vi "Core-Timer.vi"(7 "Ticks Begin In [ms]":u64, 8 "error in (no error)":errorcluster, 11 "Engine in":refnum<class "Engine.lvclass">) -> (0 "error out":errorcluster, 3 "Engine out":refnum<class "Engine.lvclass">, 5 "Ticks Begin Out [ms]":u64)   [LabVIEW 2020, in "GLF.lvlib" / "Engine.lvclass"]
uses:
  Engine.lvclass
  Engine.lvclass/Engine.ctl
  <vilib>/Saukko/LV SDL3/Sources/SDL3/Timer/Timer.lvlib
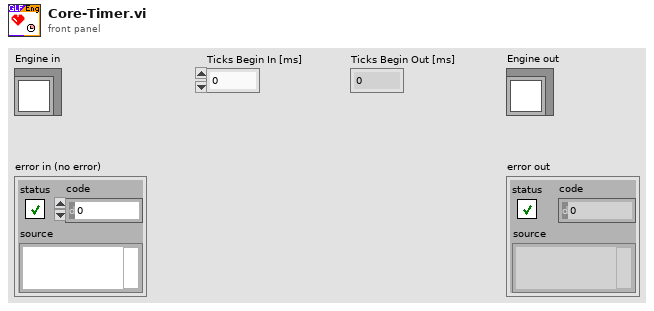
[diagram p1: front panel]
types:
  T1 = typedef "GLF.lvlib/Engine.lvclass/DVR--cluster.ctl" = cluster{"CMD Queue":T2, "Config":T3, "Ctxt":T5, "Metrics":T6, "Debug":T7, "ID To Window":map{T9, refnum<class "Window.lvclass">}, "Window To Handle":map{refnum<class "Window.lvclass">, i64}, "Event Interface":refnum<class "EngineEventInterface.lvclass">}
  T2 = typedef "GLF.lvlib/Engine.lvclass/Command--queue.ctl" = refnum<queue>
  T3 = typedef "GLF.lvlib/Engine.lvclass/Config--cluster.ctl" = cluster{"Quit On Last Window Closed":bool, "VSync":T4, "FPS Target":dbl}
  T4 = typedef "GLF.lvlib/Engine.lvclass/VSync--enum.ctl" = enum16{"Disabled", "Enabled", "Adaptative"}
  T5 = typedef "GLF.lvlib/Engine.lvclass/Context--cluster.ctl" = cluster{"VSync Enabled":bool}
  T6 = typedef "GLF.lvlib/Engine.lvclass/Metrics--cluster.ctl" = cluster{"Uptime [ms]":u64, "Loop Time [ms]":u64, "Timer [ns]":u64, "Poll Events [ns]":u64, "Dequeue CMD [ns]":u64, "Update Layout [ns]":u64, "Render [ns]":u64}
  T7 = typedef "GLF.lvlib/Engine.lvclass/Debug--cluster.ctl" = cluster{"Unhandled Events":map{T8, u64}}
  T8 = typedef "SDL3.lvlib/Events.lvlib/EventType--enum.ctl" = enum16{"LV_NONE", "LV_UNSUPPORTED", "SDL_EVENT_QUIT", "SDL_EVENT_LOCALE_CHANGED", "SDL_EVENT_SYSTEM_THEME_CHANGED", "SDL_EVENT_DISPLAY_ORIENTATION", "SDL_EVENT_DISPLAY_ADDED", "SDL_EVENT_DISPLAY_REMOVED", "SDL_EVENT_DISPLAY_MOVED", "SDL_EVENT_DISPLAY_DESKTOP_MODE_CHANGED", "SDL_EVENT_DISPLAY_CURRENT_MODE_CHANGED", "SDL_EVENT_DISPLAY_CONTENT_SCALE_CHANGED", "SDL_EVENT_WINDOW_SHOWN", "SDL_EVENT_WINDOW_HIDDEN", "SDL_EVENT_WINDOW_EXPOSED", "SDL_EVENT_WINDOW_MOVED", "SDL_EVENT_WINDOW_RESIZED", "SDL_EVENT_WINDOW_PIXEL_SIZE_CHANGED", "SDL_EVENT_WINDOW_METAL_VIEW_RESIZED", "SDL_EVENT_WINDOW_MINIMIZED", "SDL_EVENT_WINDOW_MAXIMIZED", "SDL_EVENT_WINDOW_RESTORED", "SDL_EVENT_WINDOW_MOUSE_ENTER", "SDL_EVENT_WINDOW_MOUSE_LEAVE", "SDL_EVENT_WINDOW_FOCUS_GAINED", "SDL_EVENT_WINDOW_FOCUS_LOST", "SDL_EVENT_WINDOW_CLOSE_REQUESTED", "SDL_EVENT_WINDOW_HIT_TEST", "SDL_EVENT_WINDOW_ICCPROF_CHANGED", "SDL_EVENT_WINDOW_DISPLAY_CHANGED", "SDL_EVENT_WINDOW_DISPLAY_SCALE_CHANGED", "SDL_EVENT_WINDOW_SAFE_AREA_CHANGED", "SDL_EVENT_WINDOW_OCCLUDED", "SDL_EVENT_WINDOW_ENTER_FULLSCREEN", "SDL_EVENT_WINDOW_LEAVE_FULLSCREEN", "SDL_EVENT_WINDOW_DESTROYED", "SDL_EVENT_WINDOW_HDR_STATE_CHANGED", "SDL_EVENT_KEY_DOWN", "SDL_EVENT_KEY_UP", "SDL_EVENT_TEXT_EDITING", "SDL_EVENT_TEXT_INPUT", "SDL_EVENT_KEYMAP_CHANGED", "SDL_EVENT_KEYBOARD_ADDED", "SDL_EVENT_KEYBOARD_REMOVED", "SDL_EVENT_TEXT_EDITING_CANDIDATES", "SDL_EVENT_MOUSE_MOTION", "SDL_EVENT_MOUSE_BUTTON_DOWN", "SDL_EVENT_MOUSE_BUTTON_UP", "SDL_EVENT_MOUSE_WHEEL", "SDL_EVENT_MOUSE_ADDED", "SDL_EVENT_MOUSE_REMOVED", "SDL_EVENT_JOYSTICK_AXIS_MOTION", "SDL_EVENT_JOYSTICK_BALL_MOTION", "SDL_EVENT_JOYSTICK_HAT_MOTION", "SDL_EVENT_JOYSTICK_BUTTON_DOWN", "SDL_EVENT_JOYSTICK_BUTTON_UP", "SDL_EVENT_JOYSTICK_ADDED", "SDL_EVENT_JOYSTICK_REMOVED", "SDL_EVENT_JOYSTICK_BATTERY_UPDATED", "SDL_EVENT_JOYSTICK_UPDATE_COMPLETE", "SDL_EVENT_GAMEPAD_AXIS_MOTION", "SDL_EVENT_GAMEPAD_BUTTON_DOWN", "SDL_EVENT_GAMEPAD_BUTTON_UP", "SDL_EVENT_GAMEPAD_ADDED", "SDL_EVENT_GAMEPAD_REMOVED", "SDL_EVENT_GAMEPAD_REMAPPED", "SDL_EVENT_GAMEPAD_TOUCHPAD_DOWN", "SDL_EVENT_GAMEPAD_TOUCHPAD_MOTION", "SDL_EVENT_GAMEPAD_TOUCHPAD_UP", "SDL_EVENT_GAMEPAD_SENSOR_UPDATE", "SDL_EVENT_GAMEPAD_UPDATE_COMPLETE", "SDL_EVENT_GAMEPAD_STEAM_HANDLE_UPDATED", "SDL_EVENT_FINGER_DOWN", "SDL_EVENT_FINGER_UP", "SDL_EVENT_FINGER_MOTION", "SDL_EVENT_CLIPBOARD_UPDATE", "SDL_EVENT_DROP_FILE", "SDL_EVENT_DROP_TEXT", "SDL_EVENT_DROP_BEGIN", "SDL_EVENT_DROP_COMPLETE", "SDL_EVENT_DROP_POSITION", "SDL_EVENT_AUDIO_DEVICE_ADDED", "SDL_EVENT_AUDIO_DEVICE_REMOVED", "SDL_EVENT_AUDIO_DEVICE_FORMAT_CHANGED", "SDL_EVENT_SENSOR_UPDATE", "SDL_EVENT_PEN_PROXIMITY_IN", "SDL_EVENT_PEN_PROXIMITY_OUT", "SDL_EVENT_PEN_DOWN", "SDL_EVENT_PEN_UP", "SDL_EVENT_PEN_BUTTON_DOWN", "SDL_EVENT_PEN_BUTTON_UP", "SDL_EVENT_PEN_MOTION", "SDL_EVENT_PEN_AXIS", "SDL_EVENT_CAMERA_DEVICE_ADDED", "SDL_EVENT_CAMERA_DEVICE_REMOVED", "SDL_EVENT_CAMERA_DEVICE_APPROVED", "SDL_EVENT_CAMERA_DEVICE_DENIED", "SDL_EVENT_RENDER_TARGETS_RESET", "SDL_EVENT_RENDER_DEVICE_RESET", "SDL_EVENT_POLL_SENTINEL", "SDL_EVENT_USER"}
  T9 = typedef "SDL3.lvlib/Video.lvlib/WindowID--integer.ctl" = u32
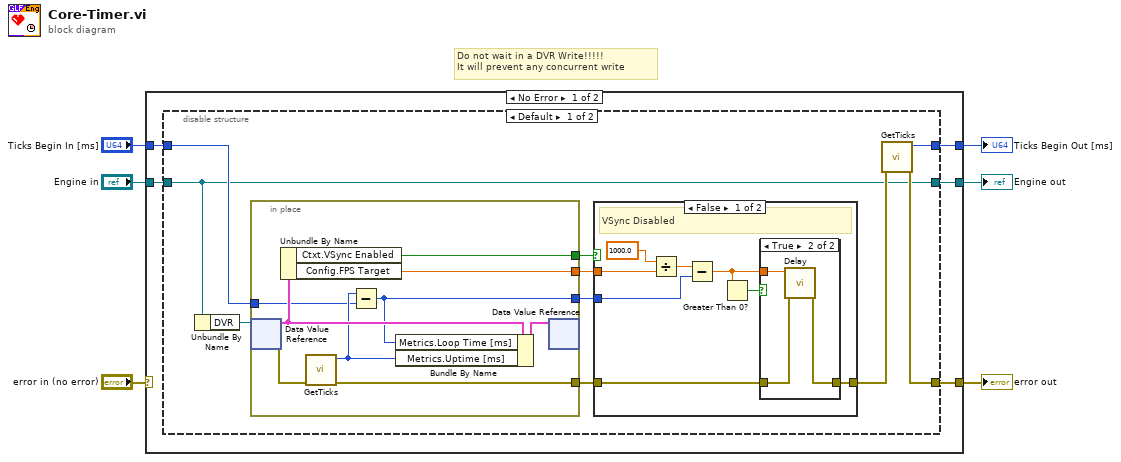
[diagram p0: block diagram]
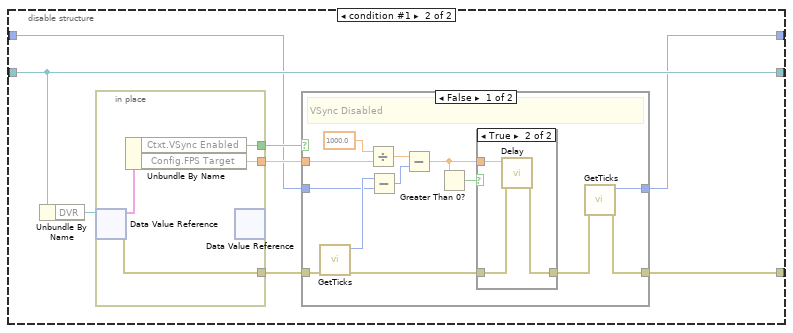
[diagram p4: hidden frame]
diagram:
  # "Do not wait in a DVR Write!!!!!\nIt will prevent any concurrent write"
  n1 = case shown="No Error" "error in (no error)" {
    selector: "error in (no error)" -> [_ w77]
    tunnel: "Engine in" -> [w8 w76]
    tunnel: [w11 w77] -> w5
    tunnel: [w7 w76] -> w4
    tunnel: "Ticks Begin In [ms]" -> [w10 w75]
    tunnel: [w9 w75] -> w1
    frame No Error {
      n2 = disable-structure shown="Default" {
        disable-tunnel: [w21 w44] -> w11
        disable-tunnel: w10 -> [w15 w46]
        disable-tunnel: [w13 w45] -> w9
        disable-tunnel: w8 -> [w12 w47]
        disable-tunnel: [w12 w47] -> w7
        frame condition #0 (active) {
          n3 = Unbundle By Name(w12) -> ("DVR"=w20:refnum<data-value>)
          n4 = in-place {
            in-place-border: [w30] -> w17
            in-place-border: [w25] -> w19
            in-place-border: [w24] -> w18
            in-place-border: [w23] -> w16
            in-place-border: w15 -> [w22]
            n5 = in-place-dvr #1(w20) -> (w27:T1, w28:errorcluster)
            n6 = Unbundle By Name(w27) -> ("Ctxt.VSync Enabled"=w23:bool, "Config.FPS Target"=w25:dbl)
            n7 = call <vilib>:"GetTicks.vi"("No Error"=w28) -> ("error out"=w30:errorcluster, "Ticks [ms]"=w26:u64)  [unwired: 9 in]
            n8 = Subtract(x=w26, y=w22) -> (x-y=w24:u64)
            n9 = Bundle By Name(cluster=w27, "Metrics.Loop Time [ms]"=w24, "Metrics.Uptime [ms]"=w26) -> (w29:T1)
            n10 = in-place-dvr #1(w29) -> ()  [unwired: 2 out]
          }
          n11 = case shown="False" w16 {
            tunnel: w19 -> [w38 _]
            tunnel: w18 -> [w35 _]
            tunnel: w17 -> [w34 w43]
            tunnel: [w31 w43] -> w14
            frame False {
              # "VSync Disabled"
              n12 = Divide(x=1000.0, y=w38) -> (x/y=w36:dbl)
              n13 = Subtract(x=w36, y=w35) -> (x-y=w33:dbl)
              n14 = Greater Than 0?(x=w33) -> (x > 0?=w32:bool)
              n15 = case shown="True" w32 {
                tunnel: w34 -> [w39 w42]
                tunnel: [w39 w41] -> w31
                tunnel: w33 -> [_ w40]
                frame False {
                }
                frame True {
                  n16 = call <vilib>:"Delay.vi"("No Error"=w42, "ms"=w40) -> ("error out"=w41:errorcluster)  [unwired: 9 in]
                }
              }
            }
            frame True {
              # "Render present will take care of waiting for us"
              # "VSync Enabled"
            }
          }
          n17 = call <vilib>:"GetTicks.vi"("No Error"=w14) -> ("error out"=w21:errorcluster, "Ticks [ms]"=w13:u64)  [unwired: 9 in]
        }
        frame condition #1 {
          n18 = Unbundle By Name(w47) -> ("DVR"=w51:refnum<data-value>)
          n19 = in-place {
            in-place-border: [w52] -> w49
            in-place-border: [w55] -> w50
            in-place-border: [w54] -> w48
            n20 = in-place-dvr #2(w51) -> (w53:T1, w52:errorcluster)
            n21 = Unbundle By Name(w53) -> ("Ctxt.VSync Enabled"=w54:bool, "Config.FPS Target"=w55:dbl)
            n22 = in-place-dvr #2() -> ()  [unwired: 1 in, 2 out]
          }
          n23 = case shown="False" w48 {
            tunnel: w50 -> [w68 _]
            tunnel: w46 -> [w60 w73]
            tunnel: w49 -> [w62 w74]
            tunnel: [w57 w74] -> w44
            tunnel: [w56 w73] -> w45
            frame False {
              # "VSync Disabled"
              n24 = call <vilib>:"GetTicks.vi"("No Error"=w62) -> ("error out"=w61:errorcluster, "Ticks [ms]"=w63:u64)  [unwired: 9 in]
              n25 = Divide(x=1000.0, y=w68) -> (x/y=w66:dbl)
              n26 = Subtract(x=w63, y=w60) -> (x-y=w59:u64)
              n27 = Subtract(x=w66, y=w59) -> (x-y=w65:dbl)
              n28 = Greater Than 0?(x=w65) -> (x > 0?=w64:bool)
              n29 = case shown="True" w64 {
                tunnel: w61 -> [w69 w72]
                tunnel: [w69 w71] -> w58
                tunnel: w65 -> [_ w70]
                frame False {
                }
                frame True {
                  n30 = call <vilib>:"Delay.vi"("No Error"=w72, "ms"=w70) -> ("error out"=w71:errorcluster)  [unwired: 9 in]
                }
              }
              n31 = call <vilib>:"GetTicks.vi"("No Error"=w58) -> ("error out"=w57:errorcluster, "Ticks [ms]"=w56:u64)  [unwired: 9 in]
            }
            frame True {
              # "Render present will take care of waiting for us"
              # "VSync Enabled"
            }
          }
        }
      }
    }
    frame Error {
    }
  }
  "error out" <- w5
  "Engine out" <- w4
  "Ticks Begin Out [ms]" <- w1
